vi "IP Changer.vi"() -> ()   [LabVIEW 2015]
uses:
  NotifyIcon VIS/TypeDefs/NotifyIcon Events.ctl
  NotifyIcon VIS/TypeDefs/NotifyIcon Event Registration Actions.ctl
  <vilib>/Utility/miscctls.llb/LVRectTypeDef.ctl
panel:
  in  "Text":string="Um novo dispositivo foi conectado a porta de rede.\nClique para configurar um novo IP."
  in  "Title":string="Novo dispositivo conectado"
  in  "Icon (None)":i32(ring)=1 items=["None", "Info", "Warning", "Error"]
  in  "Tab Control":enum32{"Your IP", "Fixed Config"}(tab)
  out "Result":string
  in  "Your IP":cluster{"DHCP":bool, "FIXED":bool}
  in  "IP":string="0.0.0.0"
  in  "Mask":string="255.255.255.0"
  in  "Gateway":string="0.0.0.0"
  in  "Adapter":string="Local Area Connection"
  # "Enter your desired fixed IP configuration"
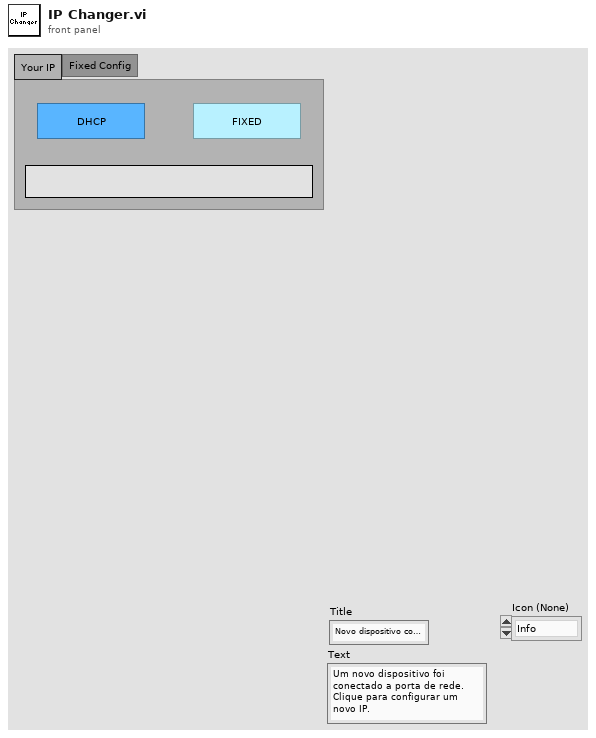
[diagram p1: front panel]
types:
  T1 = typedef "NotifyIcon Event Registration Actions.ctl" = enum16{"Initial Event Registration", "Add to Event Registration", "Destroy Events and Re-register"}
  T2 = typedef "NotifyIcon Events.ctl" = enum16{"BalloonTipClicked", "BalloonTipClosed", "BalloonTipShown", "Click", "Disposed", "DoubleClick", "MouseClick", "MouseDoubleClick", "MouseDown", "MouseMove", "MouseUp", "MenuItemClick", "MenuItemSelect"}
  T3 = enum32{"Invalid", "Standard", "Closed", "Hidden", "Minimized", "Maximized"}
  T4 = typedef "NotifyIcon Event Data.ctl" = cluster{"NotifyIcon Event":T2, "Data String":string}
  T5 = typedef "LVRectTypeDef.ctl" = cluster{"Left":i16, "Top":i16, "Right":i16, "Bottom":i16}
  T6 = cluster{"Name":string, "IP":string, "Mask":string, "Gateway":string, "Front Panel.PanelBounds":T5}
  T7 = enum16{"open", "replace", "create", "open or create", "replace or create", "replace or create with confirmation"}
  T8 = cluster{"Adapter":string, "IP":string, "Mask":string, "Gateway":string, "Front Panel.PanelBounds":T5}
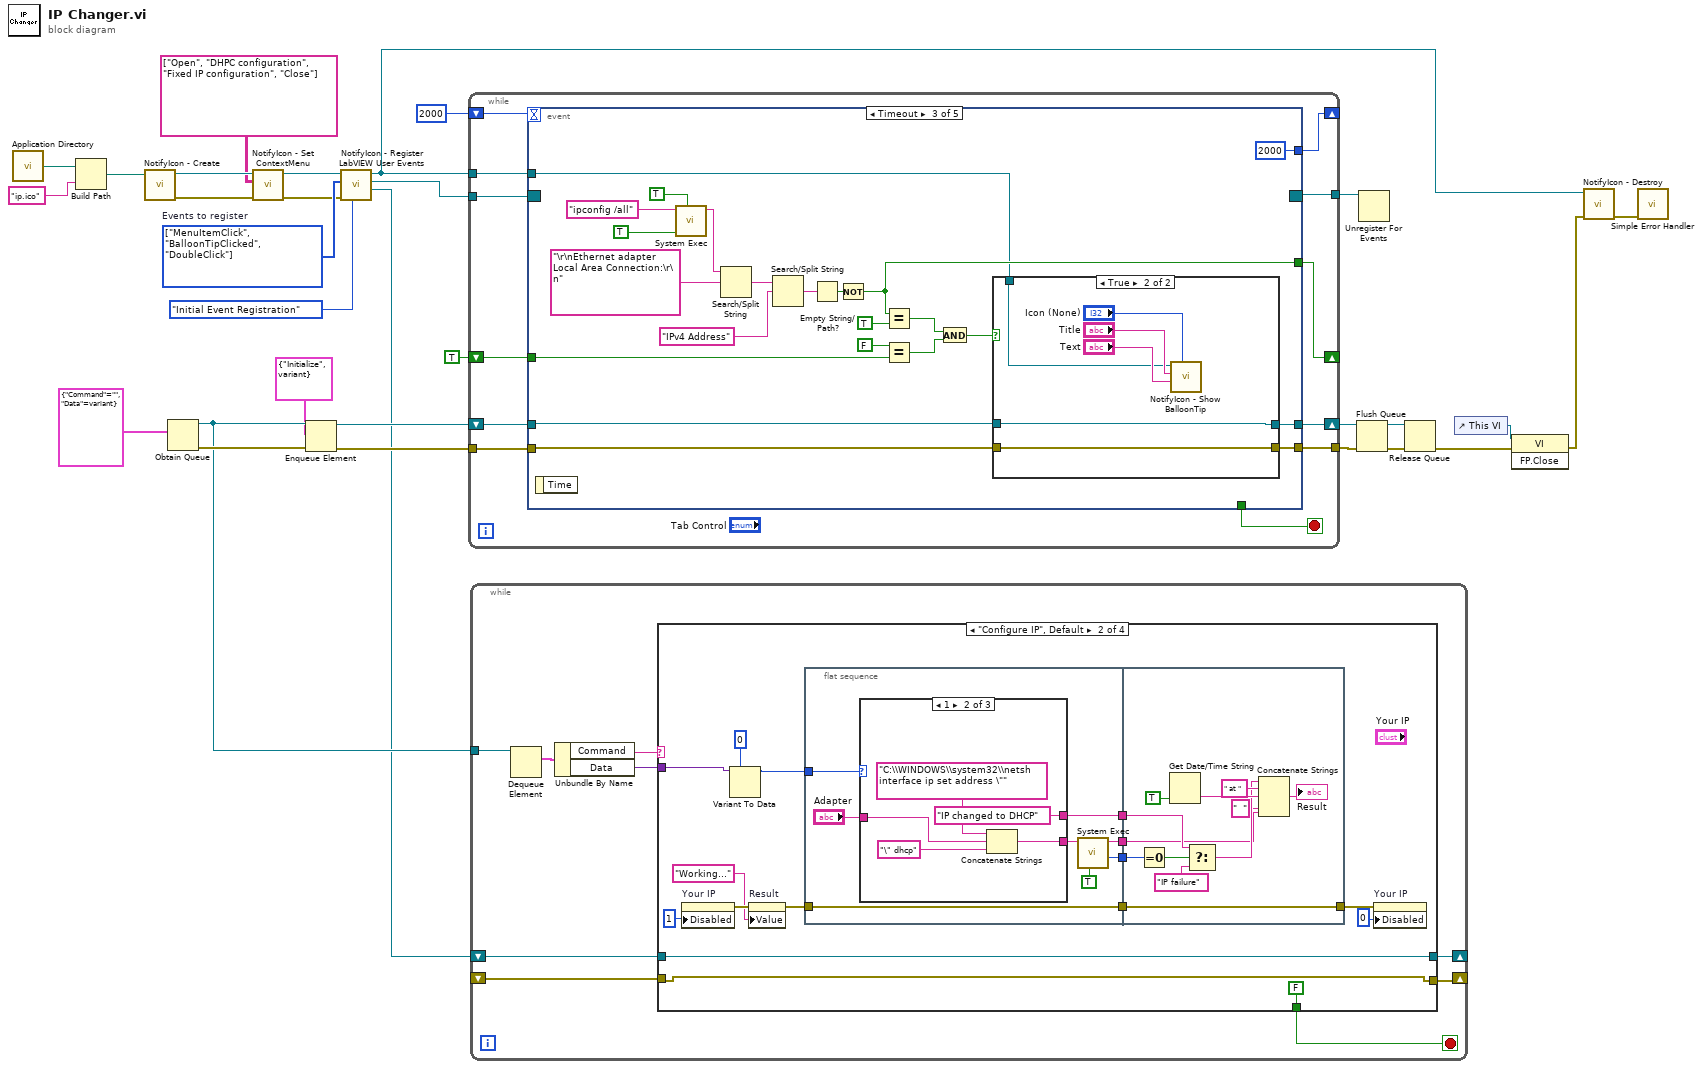
[diagram p0: block diagram]
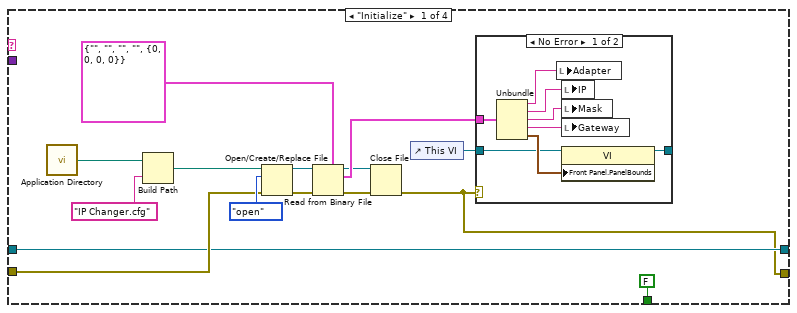
[diagram p2: hidden frame]
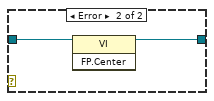
[diagram p3: hidden frame]
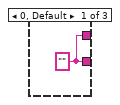
[diagram p4: hidden frame]
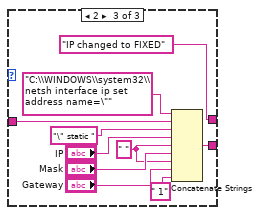
[diagram p5: hidden frame]
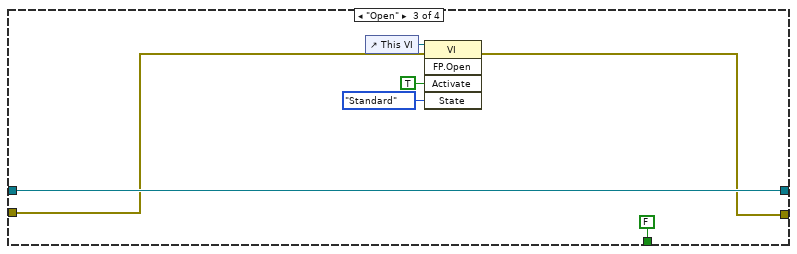
[diagram p6: hidden frame]
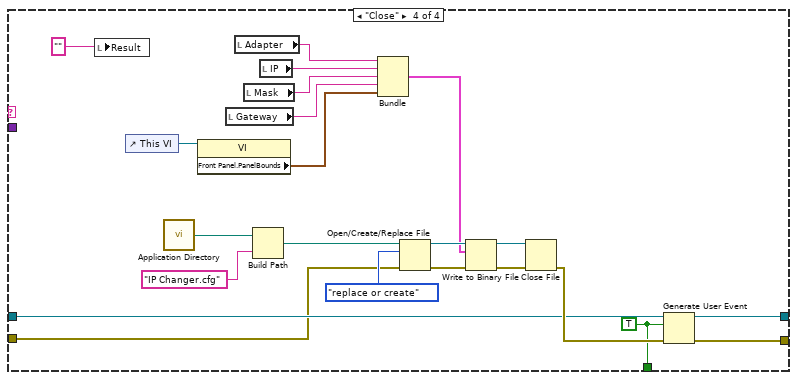
[diagram p7: hidden frame]
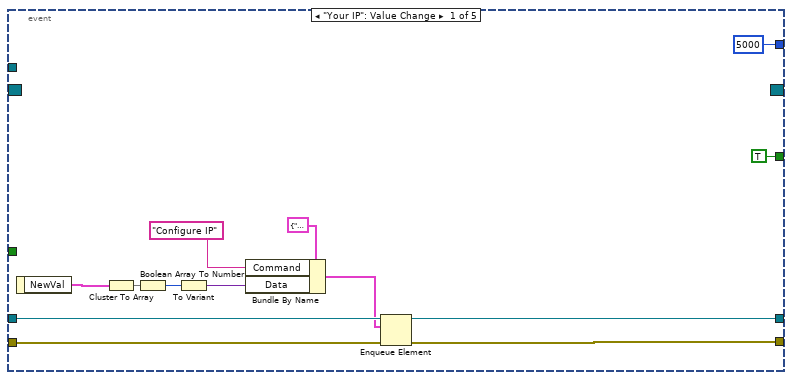
[diagram p8: hidden frame]
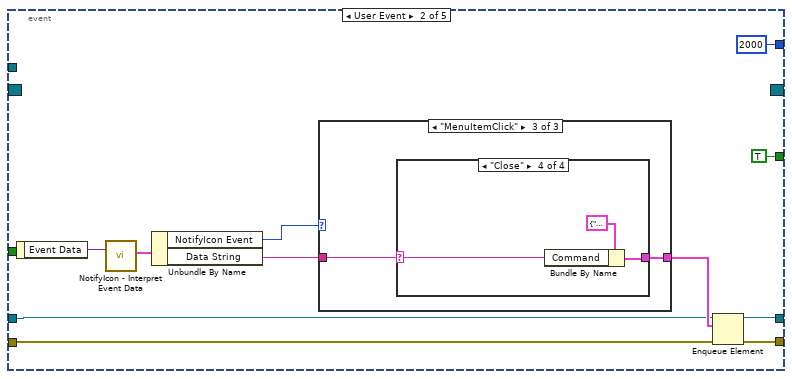
[diagram p9: hidden frame]
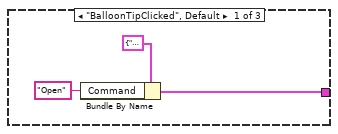
[diagram p10: hidden frame]
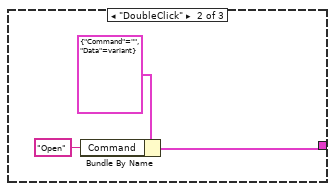
[diagram p11: hidden frame]
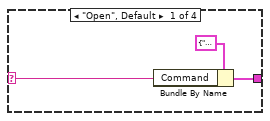
[diagram p12: hidden frame]
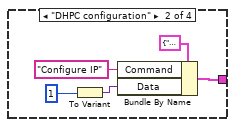
[diagram p13: hidden frame]
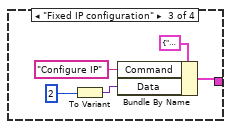
[diagram p14: hidden frame]
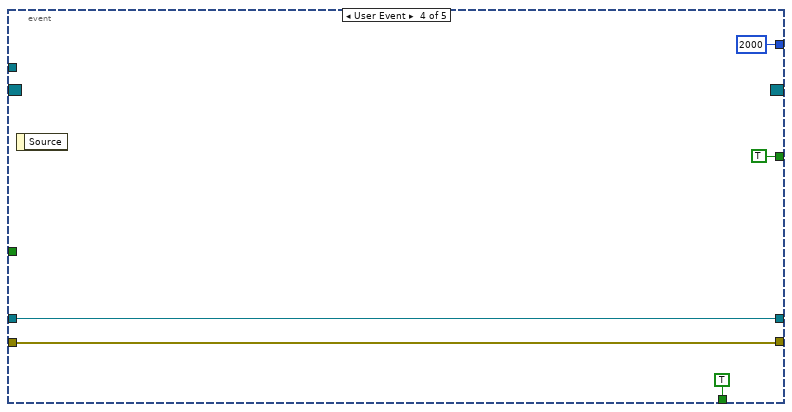
[diagram p16: hidden frame]
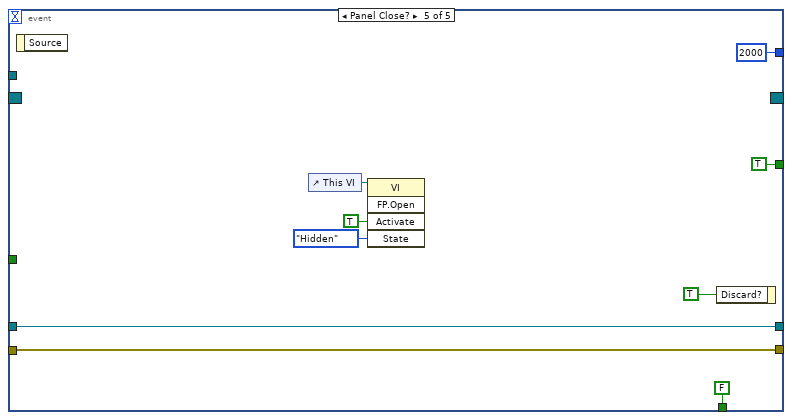
[diagram p17: hidden frame]
diagram:
  w28 = T2[] [enum."MenuItemClick", enum."BalloonTipClicked", enum."DoubleClick"] items=["BalloonTipClicked", "BalloonTipClosed", "BalloonTipShown", "Click", "Disposed", "DoubleClick", "MouseClick", "MouseDoubleClick", "MouseDown", "MouseMove", "MouseUp", "MenuItemClick", "MenuItemSelect"]  # Events to register
  n1 = call <vilib>:"Application Directory.vi"() -> ("Application Directory"=w20:path)
  n2 = Build Path(base path=w20, name or relative path="ip.ico") -> (appended path=w19:path)
  n3 = call "NotifyIcon - Create.vi"("Icon File Path"=w19) -> ("error out"=w26:errorcluster, "NotifyIcon reference"=w24:refnum<k24>)  [unwired: 9 in]
  n4 = Obtain Queue(element data type=cluster{"Command":string, "Data":variant} {"Command"="", "Data"=variant}) -> (queue out=w11:refnum<queue>, error out=w14:errorcluster)  [unwired: 4 in, 1 out]
  n5 = call "NotifyIcon - Set ContextMenu.vi"("error in"=w26, "Context Menu"=string[][] [["Open"], ["DHPC configuration"], ["Fixed IP configuration"], ["Close"]], "NotifyIcon reference in"=w24) -> ("error out"=w25:errorcluster, "NotifyIcon reference out"=w23:refnum<k24>)  [unwired: 7 in]
  n6 = Enqueue Element(queue=w11, element=cluster{"Command":string, "Data":variant} {"Command"="Initialize", "Data"=variant}, error in (no error)=w14) -> (queue out=w13:refnum<queue>, error out=w12:errorcluster)  [unwired: 1 in, 1 out]
  n7 = call "NotifyIcon - Register LabVIEW User Events.vi"("Action"=NotifyIcon_Event_Registration_Actions."Initial Event Registration", "error in"=w25, "Events to register"=w28, "NotifyIcon reference in"=w23) -> ("user event - Close application"=w3:refnum<user-event>, "Event Registration Refnum"=w29:refnum<event-registration>, "NotifyIcon reference out"=w17:refnum<k24>)  [unwired: 4 in, 1 out]
  n8 = while {
    tunnel: [w41] -> w8
    tunnel: w17 -> [w33]
    tunnel: w29 -> [w40]
    tunnel: w12 -> [w38]
    shift-right: [w37] -> w9
    shift-left: w13 -> [w39]
    tunnel: [w36] -> w4
    shift-right: [w35] -> _
    shift-left: TRUE -> [w34]
    shift-right: [w31] -> _
    shift-left: 2000 -> [w32]
    stop <- w42 stop-if-true
    n9 = event shown="[2] Timeout" {
      selector: w40 -> [_ _ _ _ _]
      dyn-events: [_ _ _ _ _] -> w36
      timeout: w32 -> [_ _ _ _ _]
      tunnel: [_ _ _ TRUE ("Discard?") FALSE ("Discard?")] -> w42
      tunnel: [w45 w61 w95 w123 w128] -> w41
      tunnel: w39 -> [w53 w63 w94 w124 w129]
      tunnel: w38 -> [w52 w60 w93 w123 w128]
      tunnel: [w46 w62 w96 w124 w129] -> w37
      tunnel: [TRUE TRUE w103 TRUE TRUE] -> w35
      tunnel: w34 -> [_ _ w101 _ _]
      tunnel: w33 -> [_ _ w92 _ _]
      tunnel: [5000 2000 2000 2000 2000] -> w31
      event "Your IP": Value Change {
        n10 = event-data() -> ("NewVal"=w54:cluster{"DHCP":bool, "FIXED":bool})  [unwired: 1 in]
        n11 = Cluster To Array(cluster=w54) -> (array=w55:bool[])
        n12 = Boolean Array To Number(Boolean array=w55) -> (number=w51:u32)
        n13 = To Variant(anything=w51) -> (Variant=w50:variant)
        n14 = Bundle By Name(cluster=cluster{"Command":string, "Data":variant} {"Command"="", "Data"=variant}, "Command"="Configure IP", "Data"=w50) -> (w47:cluster{"Command":string, "Data":variant})
        n15 = Enqueue Element(queue=w53, element=w47, error in (no error)=w52) -> (queue out=w46:refnum<queue>, error out=w45:errorcluster)  [unwired: 1 in, 1 out]
      }
      event User Event {
        n16 = event-data() -> ("Event Data"=w65:variant)  [unwired: 1 in]
        n17 = call "NotifyIcon - Interpret Event Data.vi"("NotifyIcon Event Data"=w65) -> ("NotifyIcon Event Data"=w66:T4)  [unwired: 9 in, 1 out]
        n18 = Unbundle By Name(w66) -> ("NotifyIcon Event"=w56:T2, "Data String"=w59:string)
        n19 = case shown="\"MenuItemClick\"" w56 {
          tunnel: [w68 w70 w74] -> w64
          tunnel: w59 -> [_ _ w73]
          frame "BalloonTipClicked", Default {
            n20 = Bundle By Name(cluster=cluster{"Command":string, "Data":variant} {"Command"="", "Data"=variant}, "Command"="Open") -> (w68:cluster{"Command":string, "Data":variant})
          }
          frame "DoubleClick" {
            n21 = Bundle By Name(cluster=cluster{"Command":string, "Data":variant} {"Command"="", "Data"=variant}, "Command"="Open") -> (w70:cluster{"Command":string, "Data":variant})
          }
          frame "MenuItemClick" {
            n22 = case shown="\"Close\"" w73 {
              selector: w73 -> [w75 _ _ w88]
              tunnel: [w76 w81 w83 w89] -> w74
              frame "Open", Default {
                n23 = Bundle By Name(cluster=cluster{"Command":string, "Data":variant} {"Command"="", "Data"=variant}, "Command"=w75) -> (w76:cluster{"Command":string, "Data":variant})
              }
              frame "DHPC configuration" {
                n24 = To Variant(anything=1) -> (Variant=w79:variant)
                n25 = Bundle By Name(cluster=cluster{"Command":string, "Data":variant} {"Command"="", "Data"=variant}, "Command"="Configure IP", "Data"=w79) -> (w81:cluster{"Command":string, "Data":variant})
              }
              frame "Fixed IP configuration" {
                n26 = To Variant(anything=2) -> (Variant=w85:variant)
                n27 = Bundle By Name(cluster=cluster{"Command":string, "Data":variant} {"Command"="", "Data"=variant}, "Command"="Configure IP", "Data"=w85) -> (w83:cluster{"Command":string, "Data":variant})
              }
              frame "Close" {
                n28 = Bundle By Name(cluster=cluster{"Command":string, "Data":variant} {"Command"="", "Data"=variant}, "Command"=w88) -> (w89:cluster{"Command":string, "Data":variant})
              }
            }
          }
        }
        n29 = Enqueue Element(queue=w63, element=w64, error in (no error)=w60) -> (queue out=w62:refnum<queue>, error out=w61:errorcluster)  [unwired: 1 in, 1 out]
      }
      event Timeout {
        n30 = event-data() -> ()  [unwired: 1 in, 1 out]
        n31 = call <vilib>:"System Exec.vi"("run minimized? (F)"=TRUE, "wait until completion? (T)"=TRUE, "command line"="ipconfig /all") -> ("standard output"=w111:string)  [unwired: 5 in, 3 out]
        n32 = Search/Split String(string=w111, search string/char (-)="\r\nEthernet adapter Local Area Connection:\r\n") -> (match + rest of string=w109:string)  [unwired: 1 in, 2 out]
        n33 = Search/Split String(string=w109, search string/char (-)="IPv4 Address") -> (match + rest of string=w107:string)  [unwired: 1 in, 2 out]
        n34 = Empty String/Path?(string/path=w107) -> (empty?=w106:bool)
        n35 = Not(x=w106) -> (.not. x?=w103:bool)
        n36 = Equal?(x=w103, y=TRUE) -> (x = y?=w98:bool)
        n37 = Equal?(x=FALSE ("y"), y=w101) -> (x = y?=w99:bool)
        n38 = And(x=w98, y=w99) -> (x .and. y?=w97:bool)
        n39 = case shown="True" w97 {
          tunnel: [w114 w117] -> w96
          tunnel: [w113 w116] -> w95
          tunnel: w94 -> [w114 w117]
          tunnel: w93 -> [w113 w116]
          tunnel: w92 -> [_ w115]
          frame False {
          }
          frame True {
            n40 = call "NotifyIcon - Show BalloonTip.vi"("Icon (None)"="Icon (None)", "Text"="Text", "Title"="Title", "NotifyIcon reference in"=w115) -> ()  [unwired: 6 in, 2 out]
          }
        }
      }
      event User Event {
        n41 = event-data() -> ()  [unwired: 1 in, 1 out]
      }
      event Panel Close? {
        n42 = event-data() -> ()  [unwired: 1 in, 1 out]
        n43 = control-ref of="This VI"() -> (w133:refnum<vi>)
        n44 = invoke class="VI" method="FP.Open"(reference=w133, "Activate"=TRUE ("Activate?"), "State"=T3."Hidden") -> ()  [unwired: 2 in, 5 out]
        n45 = event-data("Discard?"=TRUE) -> ()  [unwired: 1 in, 1 out]
      }
    }
  }
  n46 = while {
    tunnel: w11 -> [w143]
    shift-right: [w138] -> _
    shift-left: w3 -> [w139]
    shift-right: [w137] -> _
    shift-left: _ -> [w135]
    stop <- w136 stop-if-true
    n47 = Dequeue Element(queue=w143) -> (element=w142:cluster{"Command":string, "Data":variant})  [unwired: 2 in, 3 out]
    n48 = Unbundle By Name(w142) -> ("Command"=w141:string, "Data"=w140:variant)
    n49 = case shown="\"Configure IP\", Default" w141 {
      tunnel: w140 -> [_ w172 _ _]
      tunnel: w139 -> [w145 w170 w223 w232]
      tunnel: [w145 w170 w223 w231] -> w138
      tunnel: [w144 w169 w221 w230] -> w137
      tunnel: [FALSE ("event data") FALSE ("event data") FALSE ("event data") w229] -> w136
      tunnel: w135 -> [w146 w169 w222 w228]
      frame "Initialize" {
        n50 = call <vilib>:"Application Directory.vi"() -> ("Application Directory"=w158:path)
        n51 = Build Path(base path=w158, name or relative path="IP Changer.cfg") -> (appended path=w149:path)
        n52 = Open/Create/Replace File(file path (use dialog)=w149, error in=w146, operation (0:open)=T7."open") -> (refnum out=w151:refnum<file>, error out=w152:errorcluster)  [unwired: 3 in, 1 out]
        n53 = Read from Binary File(5:T6 {"Name"="", "IP"="", "Mask"="", "Gateway"="", "Front Panel.PanelBounds"={"Left"=0, "Top"=0, "Right"=0, "Bottom"=0}} ("output cluster"), 8:w152, 11:w151) -> (0:w154:errorcluster, 2:w155:T6, 3:w153:refnum<file>)  [unwired: 3 in, 1 out]
        n54 = Close File(refnum=w153, error in=w154) -> (error out=w144:errorcluster)  [unwired: 1 out]
        n55 = control-ref of="This VI"() -> (w157:refnum<vi>)
        n56 = case shown="No Error" w144 {
          tunnel: w155 -> [w162 _]
          tunnel: w157 -> [w160 w168]
          tunnel: [w159 w167] -> _
          frame No Error {
            n57 = Unbundle(w162) -> ("Name"=w166:string, "IP"=w165:string, "Mask"=w164:string, "Gateway"=w163:string, "Front Panel.PanelBounds"=w161:T5)
            n58 = local write "Adapter"(w166) -> ()
            n59 = local write "IP"(w165) -> ()
            n60 = local write "Mask"(w164) -> ()
            n61 = local write "Gateway"(w163) -> ()
            n62 = property class="VI"(reference=w160, "Front Panel.PanelBounds"=w161) -> (reference out=w159:refnum<vi>)  [unwired: 1 in, 1 out]
          }
          frame Error {
            n63 = invoke class="VI" method="FP.Center"(reference=w168) -> (reference out=w167:refnum<vi>)  [unwired: 2 in, 2 out]
          }
        }
      }
      frame "Configure IP", Default {
        n64 = property on="Your IP" class="Clust"("Disabled"=u8 1) -> (error out=w177:errorcluster)  [unwired: 2 in, 1 out]
        n65 = Variant To Data(type=0, Variant=w172) -> (data=w173:i32)  [unwired: 1 in, 1 out]
        n66 = property on="Result" class="Str"(error in=w177, "Value"="Working..." ("Result")) -> (error out=w176:errorcluster)  [unwired: 1 in, 1 out]
        n67 = flat-sequence {
          tunnel: w173 -> [w190]
          tunnel: w176 -> [w189]
          tunnel: [w189] -> w184
          tunnel: [w187] -> w183
          tunnel: [w186] -> w182
          tunnel: [w185] -> w181
          tunnel: w184 -> [w219]
          tunnel: [w219] -> w179
          tunnel: w183 -> [w218]
          tunnel: w182 -> [w211]
          tunnel: w181 -> [w209]
          frame #0 {
            n68 = case shown="1" w190 {
              tunnel: [w193 w195 w208] -> w191
              tunnel: "Adapter" -> [_ w197 w206]
              tunnel: [w193 "IP changed to DHCP" ("Result") "IP changed to FIXED" ("Result")] -> w186
              frame 0, Default {
                w193 = ""
              }
              frame 1 {
                n69 = Concatenate Strings("C:\\WINDOWS\\system32\\netsh interface ip set address \"" ("command line"), w197, "\" dhcp" ("command line")) -> (w195:string)
              }
              frame 2 {
                w202 = " " ("string")
                n70 = Concatenate Strings("C:\\WINDOWS\\system32\\netsh interface ip set address name=\"" ("command line"), w206, "\" static " ("command line"), "IP", w202, "Mask", w202, "Gateway", " 1" ("command line")) -> (w208:string)
              }
            }
            n71 = call <vilib>:"System Exec.vi"("run minimized? (F)"=TRUE, "command line"=w191) -> ("return code"=w187:i32, "standard output"=w185:string)  [unwired: 6 in, 2 out]
          }
          frame #1 {
            n72 = Equal To 0?(x=w218) -> (x = 0?=w217:bool)
            n73 = Get Date/Time String(want seconds? (F)=TRUE) -> (time string=w215:string)  [unwired: 2 in, 1 out]
            n74 = Select(t=w211, s=w217, f="IP failure" ("Result")) -> (s? t:f=w212:string)
            n75 = Concatenate Strings(w212, " at " ("string"), w215, "  " ("string"), w209) -> (→"Result":string)
          }
        }
        n76 = property on="Your IP" class="Clust"(error in=w179, "Disabled"=u8 0) -> ()  [unwired: 1 in, 2 out]
      }
      frame "Open" {
        n77 = control-ref of="This VI"() -> (w227:refnum<vi>)
        n78 = invoke class="VI" method="FP.Open"(reference=w227, error in=w222, "Activate"=TRUE ("Activate?"), "State"=T3."Standard") -> (error out=w221:errorcluster)  [unwired: 1 in, 4 out]
      }
      frame "Close" {
        w229 = TRUE ("event data")
        n79 = local write "Result"("" ("Result")) -> ()
        n80 = control-ref of="This VI"() -> (w244:refnum<vi>)
        n81 = call <vilib>:"Application Directory.vi"() -> ("Application Directory"=w235:path)
        n82 = property class="VI"(reference=w244) -> ("Front Panel.PanelBounds"=w243:T5)  [unwired: 1 in, 2 out]
        n83 = local read "Gateway"() -> (w245:string)
        n84 = local read "Adapter"() -> (w248:string)
        n85 = local read "Mask"() -> (w246:string)
        n86 = Build Path(base path=w235, name or relative path="IP Changer.cfg") -> (appended path=w241:path)
        n87 = local read "IP"() -> (w247:string)
        n88 = Bundle("Adapter"=w248, "IP"=w247, "Mask"=w246, "Gateway"=w245, "Front Panel.PanelBounds"=w243) -> (w234:T8)  [unwired: 1 in]
        n89 = Open/Create/Replace File(file path (use dialog)=w241, error in=w228, operation (0:open)=T7."replace or create") -> (refnum out=w240:refnum<file>, error out=w237:errorcluster)  [unwired: 3 in, 1 out]
        n90 = Write to Binary File(file (use dialog)=w240, data=w234, error in=w237) -> (refnum out=w239:refnum<file>, error out=w236:errorcluster)  [unwired: 3 in, 1 out]
        n91 = Close File(refnum=w239, error in=w236) -> (error out=w233:errorcluster)  [unwired: 1 out]
        n92 = Generate User Event(user event=w232, event data cluster=w229, error in=w233) -> (user event out=w231:refnum<user-event>, error out=w230:errorcluster)  [unwired: 1 in]
      }
    }
  }
  n93 = Flush Queue(queue=w9, error in (no error)=w8) -> (queue out=w7:refnum<queue>, error out=w6:errorcluster)  [unwired: 1 out]
  n94 = Unregister For Events(event registration refnum=w4) -> ()  [unwired: 1 in, 1 out]
  n95 = Release Queue(queue=w7, error in (no error)=w6) -> (error out=w5:errorcluster)  [unwired: 1 in, 2 out]
  n96 = control-ref of="This VI"() -> (w30:refnum<vi>)
  n97 = invoke class="VI" method="FP.Close"(reference=w30, error in=w5) -> (error out=w16:errorcluster)  [unwired: 1 in, 2 out]
  n98 = call "NotifyIcon - Destroy.vi"("error in"=w16, "NotifyIcon reference"=w17) -> ("error out"=w18:errorcluster)  [unwired: 9 in]
  n99 = call <vilib>:"Simple Error Handler.vi"("error in (no error)"=w18) -> ()  [unwired: 4 in, 5 out]
